vi "ConvertBeadPosCornerCenter.vi"(8 "Corner-based bead locations":cluster{"X":i32, "Y":i32}[](array[cluster]), 10 "ROI Size":cluster{"X":i32, "Y":i32}={"X"=200, "Y"=200}, 11 "Center-based bead locations":cluster{"X":i32, "Y":i32}[](array[cluster])) -> (0 "Center-based bead pos (out)":cluster{"X":i32, "Y":i32}[](array[cluster]), 3 "Corner-based bead pos (out)":cluster{"X":i32, "Y":i32}[](array[cluster]))   [LabVIEW 2011]
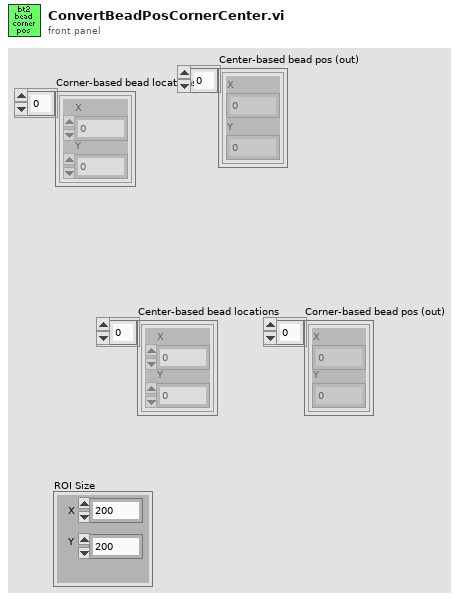
[diagram p1: front panel]
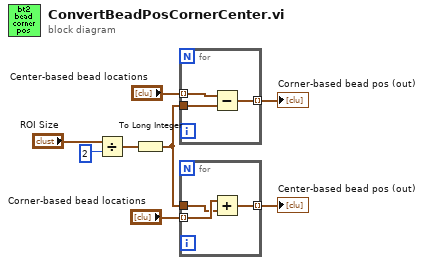
[diagram p0: block diagram]
diagram:
  n1 = Divide(x="ROI Size", y=2) -> (x/y=w7:cluster{"X":dbl, "Y":dbl})
  n2 = To Long Integer(number=w7) -> (32bit integer=w3:cluster{"X":i32, "Y":i32})
  n3 = for {
    tunnel: "Center-based bead locations" -> [w11] mode=indexing
    tunnel: w3 -> [w10]
    tunnel: [w9] -> w8 mode=indexing
    n4 = Subtract(x=w11, y=w10) -> (x-y=w9:cluster{"X":i32, "Y":i32})
  }
  "Corner-based bead pos (out)" <- w8
  n5 = for {
    tunnel: "Corner-based bead locations" -> [w14] mode=indexing
    tunnel: w3 -> [w13]
    tunnel: [w12] -> w1 mode=indexing
    n6 = Add(x=w14, y=w13) -> (x+y=w12:cluster{"X":i32, "Y":i32})
  }
  "Center-based bead pos (out)" <- w1
